vi "Throw Invalid Setting Error.vi"(7 "source vi name":string, 8 "error in (no error)":errorcluster, 9 "value":string, 10 "key":string, 11 "UDP in":refnum<class "UDP Transceiver.lvclass">) -> (0 "error out":errorcluster, 3 "UDP out":refnum<class "UDP Transceiver.lvclass">)   [LabVIEW 2017, in "UDP.lvlib" / "UDP Transceiver.lvclass"]
uses:
  UDP Transceiver.lvclass
  Errors.ctl
  <vilib>/NI/Memory Manager/Static Errors.lvlib
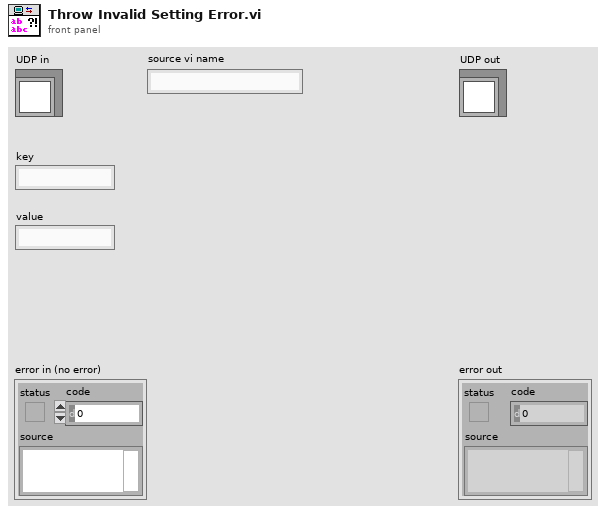
[diagram p1: front panel]
types:
  T1 = typedef "UDP.lvlib/UDP Transceiver.lvclass/Errors.ctl" = enum16{"Unknown Datagram", "Size Mismatch", "Invalid Setting"}
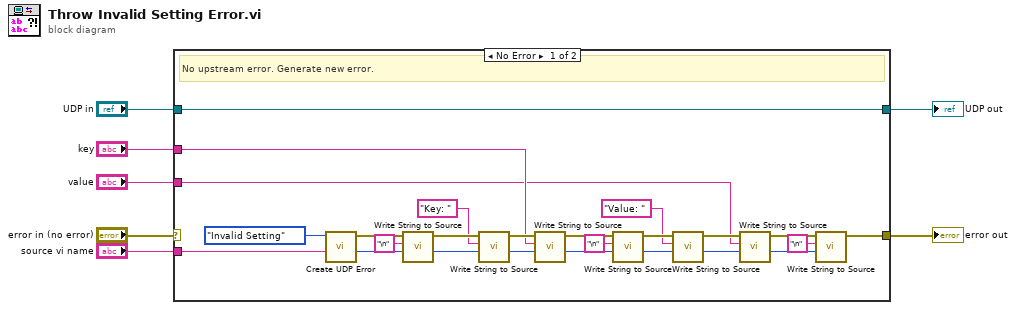
[diagram p0: block diagram]
diagram:
  n1 = case shown="No Error" "error in (no error)" {
    selector: "error in (no error)" -> [_ w33]
    tunnel: [w9 w33] -> w3
    tunnel: "UDP in" -> [w25 w34]
    tunnel: [w25 w34] -> w2
    tunnel: "value" -> [w13 _]
    tunnel: "key" -> [w22 _]
    tunnel: "source vi name" -> [w32 _]
    frame No Error {
      # "No upstream error. Generate new error."
      n2 = call "Create UDP Error.vi"("source vi name"=w32, "error"=Errors."Invalid Setting" ("Error")) -> ("offset"=w8:i32, "error out"=w29:errorcluster)  [unwired: 8 in]
      n3 = call <vilib>:"Write String to Source.vi"("offset"=w8, "string"="\n", "error in"=w29) -> ("new offset"=w27:i32, "error out"=w28:errorcluster)  [unwired: 7 in]
      n4 = call <vilib>:"Write String to Source.vi"("offset"=w27, "string"="Key: ", "error in"=w28) -> ("new offset"=w23:i32, "error out"=w24:errorcluster)  [unwired: 7 in]
      n5 = call <vilib>:"Write String to Source.vi"("offset"=w23, "string"=w22, "error in"=w24) -> ("new offset"=w19:i32, "error out"=w20:errorcluster)  [unwired: 7 in]
      n6 = call <vilib>:"Write String to Source.vi"("offset"=w19, "string"="\n", "error in"=w20) -> ("new offset"=w17:i32, "error out"=w18:errorcluster)  [unwired: 7 in]
      n7 = call <vilib>:"Write String to Source.vi"("offset"=w17, "string"="Value: ", "error in"=w18) -> ("new offset"=w15:i32, "error out"=w14:errorcluster)  [unwired: 7 in]
      n8 = call <vilib>:"Write String to Source.vi"("offset"=w15, "string"=w13, "error in"=w14) -> ("new offset"=w10:i32, "error out"=w11:errorcluster)  [unwired: 7 in]
      n9 = call <vilib>:"Write String to Source.vi"("offset"=w10, "string"="\n", "error in"=w11) -> ("error out"=w9:errorcluster)  [unwired: 7 in, 1 out]
    }
    frame Error {
      # "Upstream error. Pass through."
    }
  }
  "error out" <- w3
  "UDP out" <- w2
